vi "Defaults.vi"(8 "error in (no error)":errorcluster, 11 "MB Slave in":refnum<class "Vacon-DCGuard.lvclass">) -> (0 "error out":errorcluster, 3 "MB Slave out":refnum<class "Vacon-DCGuard.lvclass">)   [LabVIEW 2021, in "Vacon-DCGuard.lvclass"]
uses:
  Vacon-DCGuard.lvclass
  C:/Program Files (x86)/National Instruments/LabVIEW 2021/user.lib/S2 Labs/Module Framework/Modules/Modbus/Modbus Slave Base/Modbus Slave Base.lvclass
  <userlib>/S2 Labs/Modbus Toolkit/TypeDefs/MB Element.ctl
  <userlib>/S2 Labs/Modbus Toolkit/TypeDefs/Endianness Type.ctl
  <userlib>/S2 Labs/Modbus Toolkit/TypeDefs/Access Type.ctl
  <userlib>/S2 Labs/Module Framework/Modules/Modbus/Modbus Slave Base/Modbus Slave Base.lvclass/Modbus Slave Base.ctl
  <userlib>/S2 Labs/Module Framework/Modules/Modbus/Modbus Slave Base/Write MB Map.vi
  MB Slave Simulator Base/MB Slave Simulator Base.lvclass
  <userlib>/S2 Labs/Modbus Toolkit/S2L Modbus API.lvclass
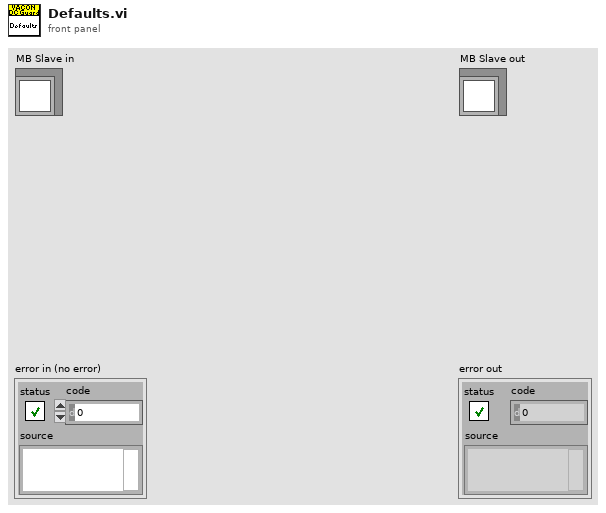
[diagram p1: front panel]
types:
  T1 = typedef "S2L Modbus API.lvclass/MB Element.ctl" = cluster{"Label":string, "Prefix":u8, "Address":u16, "Datatype":string, "Register Count":u8, "Multiplier":dbl, "Offset":dbl, "Unit":string, "Endianness":T2, "Access":T3, "LUT":string[], "Poll Rate(ms)":u16, "Mapping":cluster{"Module":string, "Channel":string}}
  T2 = typedef "Endianness Type.ctl" = enum16{"Big-Endian", "Little-Endian", "Big-Endian Byte Swap", "Little-Endian Byte Swap"}
  T3 = typedef "S2L Modbus API.lvclass/Access Type.ctl" = enum16{"R/W", "R", "W"}
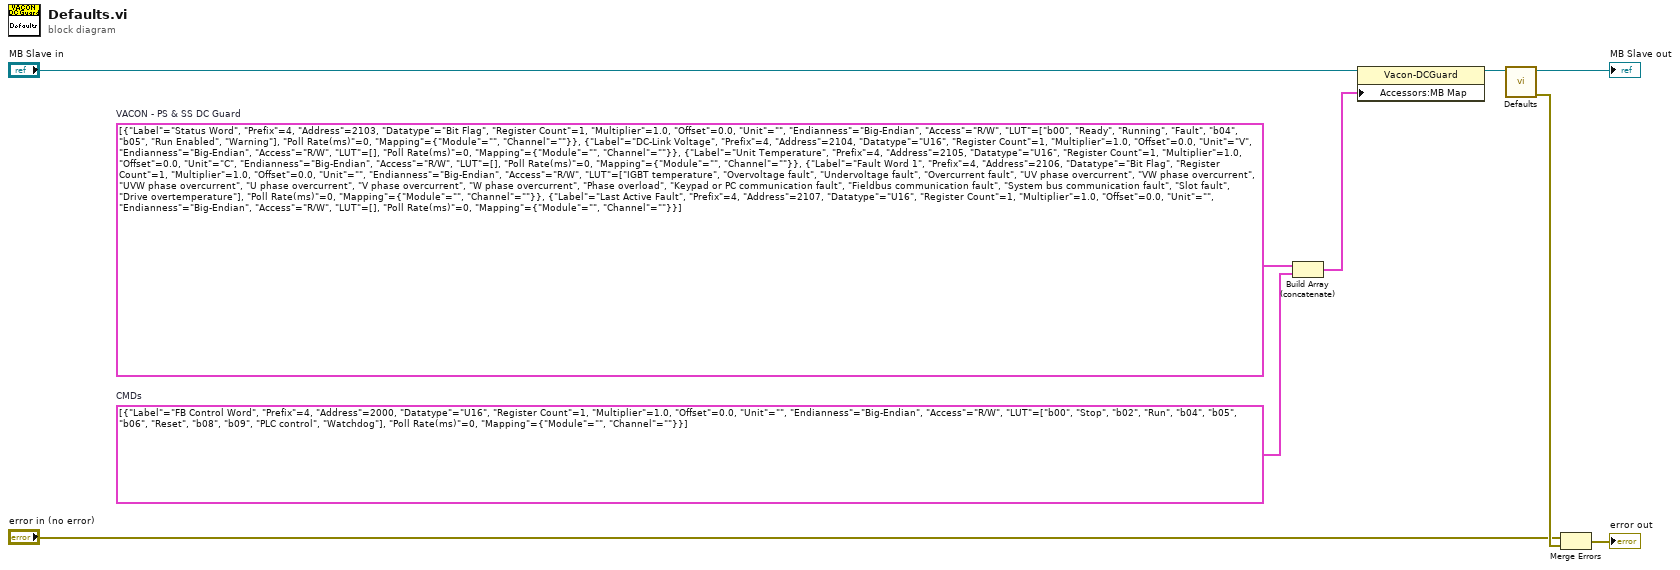
[diagram p0: block diagram]
diagram:
  w1 = T1[] [{"Label"="FB Control Word", "Prefix"=4, "Address"=2000, "Datatype"="U16", "Register Count"=1, "Multiplier"=1.0, "Offset"=0.0, "Unit"="", "Endianness"=enum."Big-Endian", "Access"=enum."R/W", "LUT"=["b00", "Stop", "b02", "Run", "b04", "b05", "b06", "Reset", "b08", "b09", "PLC control", "Watchdog"], "Poll Rate(ms)"=0, "Mapping"={"Module"="", "Channel"=""}}]  # CMDs
  w8 = T1[] [{"Label"="Status Word", "Prefix"=4, "Address"=2103, "Datatype"="Bit Flag", "Register Count"=1, "Multiplier"=1.0, "Offset"=0.0, "Unit"="", "Endianness"=enum."Big-Endian", "Access"=enum."R/W", "LUT"=["b00", "Ready", "Running", "Fault", "b04", "b05", "Run Enabled", "Warning"], "Poll Rate(ms)"=0, "Mapping"={"Module"="", "Channel"=""}}, {"Label"="DC-Link Voltage", "Prefix"=4, "Address"=2104, "Datatype"="U16", "Register Count"=1, "Multiplier"=1.0, "Offset"=0.0, "Unit"="V", "Endianness"=enum."Big-Endian", "Access"=enum."R/W", "LUT"=[], "Poll Rate(ms)"=0, "Mapping"={"Module"="", "Channel"=""}}, {"Label"="Unit Temperature", "Prefix"=4, "Address"=2105, "Datatype"="U16", "Register Count"=1, "Multiplier"=1.0, "Offset"=0.0, "Unit"="C", "Endianness"=enum."Big-Endian", "Access"=enum."R/W", "LUT"=[], "Poll Rate(ms)"=0, "Mapping"={"Module"="", "Channel"=""}}, {"Label"="Fault Word 1", "Prefix"=4, "Address"=2106, "Datatype"="Bit Flag", "Register Count"=1, "Multiplier"=1.0, "Offset"=0.0, "Unit"="", "Endianness"=enum."Big-Endian", "Access"=enum."R/W", "LUT"=["IGBT temperature", "Overvoltage fault", "Undervoltage fault", "Overcurrent fault", "UV phase overcurrent", "VW phase overcurrent", "UVW phase overcurrent", "U phase overcurrent", "V phase overcurrent", "W phase overcurrent", "Phase overload", "Keypad or PC communication fault", "Fieldbus communication fault", "System bus communication fault", "Slot fault", "Drive overtemperature"], "Poll Rate(ms)"=0, "Mapping"={"Module"="", "Channel"=""}}, {"Label"="Last Active Fault", "Prefix"=4, "Address"=2107, "Datatype"="U16", "Register Count"=1, "Multiplier"=1.0, "Offset"=0.0, "Unit"="", "Endianness"=enum."Big-Endian", "Access"=enum."R/W", "LUT"=[], "Poll Rate(ms)"=0, "Mapping"={"Module"="", "Channel"=""}}]  # VACON - PS & SS DC Guard
  n1 = Build Array (concatenate)(w8, w1) -> (w7:T1[])
  n2 = property class="Vacon-DCGuard"(reference="MB Slave in", "Accessors:MB Map"=w7) -> (reference out=w6:refnum<class "Vacon-DCGuard.lvclass">)  [unwired: 1 in, 1 out]
  n3 = call-parent "Defaults.vi"("MB Slave in"=w6) -> ("error out"=w3:errorcluster, "MB Slave out"=→"MB Slave out":refnum<class "Vacon-DCGuard.lvclass">)  [unwired: 9 in]
  n4 = Merge Errors("error in (no error)", w3) -> (→"error out":errorcluster)
